vi "validity.vi"() -> (3 "NOt valid":bool)   [LabVIEW 2023]
panel:
  out "data":timestamp
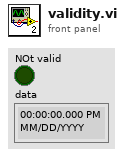
[diagram p1: front panel]
types:
  T1 = enum16{"open", "replace", "create", "open or create", "replace or create", "replace or create with confirmation"}
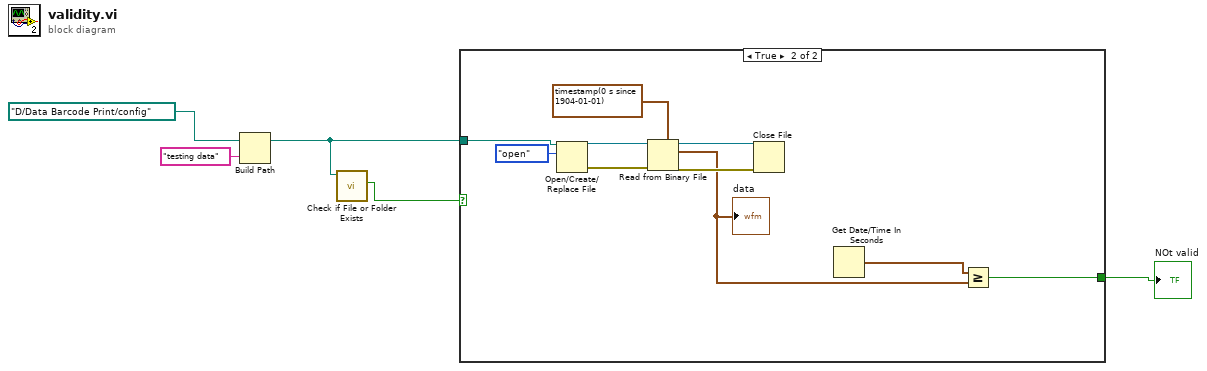
[diagram p0: block diagram]
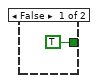
[diagram p2: hidden frame]
diagram:
  n1 = Build Path(base path=path "D:/Data Barcode Print/config" ("path"), name or relative path="testing data") -> (appended path=w3:path)
  n2 = call <vilib>:"Check if File or Folder Exists.vi"("path"=w3) -> ("file or folder exists?"=w1:bool)  [unwired: 8 in, 2 out]
  n3 = case shown="True" w1 {
    tunnel: w3 -> [_ w8]
    tunnel: [TRUE w7] -> w2
    frame False {
    }
    frame True {
      n4 = Open/Create/Replace File(file path (use dialog)=w8, operation (0:open)=T1."open") -> (refnum out=w15:refnum<file>, error out=w12:errorcluster)  [unwired: 4 in, 1 out]
      n5 = Read from Binary File(5:timestamp(0 s since 1904-01-01) ("calbration date"), 8:w12, 11:w15) -> (0:w13:errorcluster, 2:w9:timestamp, 3:w14:refnum<file>)  [unwired: 3 in, 1 out]
      "data" <- w9
      n6 = Close File(refnum=w14, error in=w13) -> ()  [unwired: 2 out]
      n7 = Get Date/Time In Seconds() -> (seconds since 1Jan1904=w16:timestamp)
      n8 = Greater Or Equal?(x=w16, y=w9) -> (x >= y?=w7:bool)
    }
  }
  "NOt valid" <- w2
